vi "2.0.0 Mutation.vi"(8 "error in":errorcluster, 11 "Device Ref in":T1 format="%.0x") -> (0 "error out":errorcluster, 3 "Device Ref out":T1 format="%.0x")   [LabVIEW 2016, in "Ballard Arinc-429 System Explorer.lvlib"]
uses:
  Ballard Arinc-429 System Explorer.lvlib
  <vilib>/NI Veristand/Custom Device API/Custom Device Item Ref.ctl
  NationalInstruments.VeriStand.SystemDefinitionAPI
  Shared/Controls and Global/Global.vi
  <vilib>/NI Veristand/Custom Device Tools/Custom Device Utility Library/NI VeriStand - Search for All Items by GUID.vi
  <vilib>/NI VeriStand/Custom Device Tools/Custom Device Utility Library/Custom Device Utility Library.lvlib
  Shared/Ballard Arinc-429 Shared.lvlib
  <vilib>/NI VeriStand/Custom Device API/Custom Device API.lvlib
  <vilib>/NI Veristand/Custom Device Offline API/Custom Device Offline API.lvlib
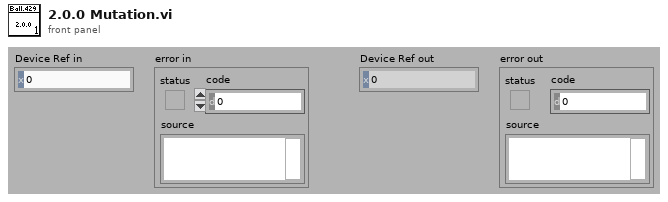
[diagram p1: front panel]
types:
  T1 = typedef "Custom Device API.lvlib/Custom Device Item Ref.ctl" = u64
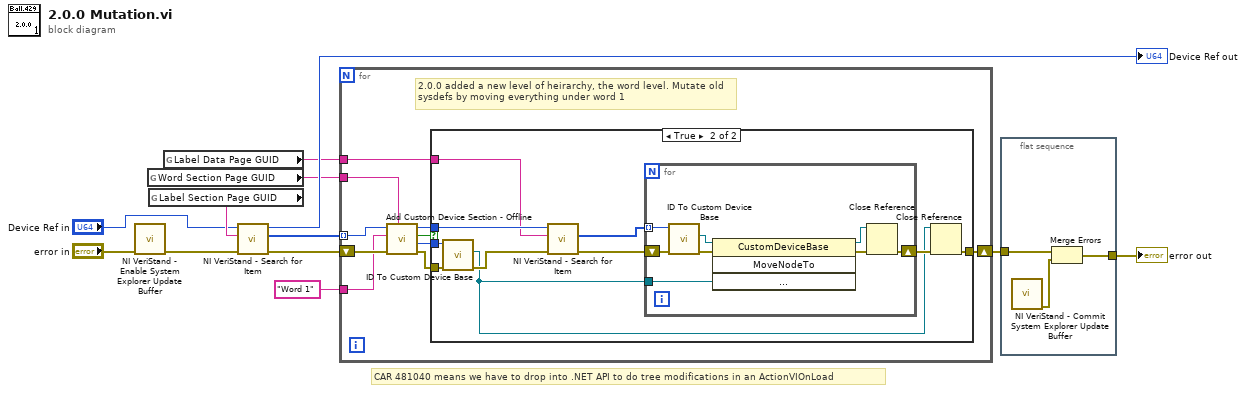
[diagram p0: block diagram]
diagram:
  # "CAR 481040 means we have to drop into .NET API to do tree modifications in an ActionVIOnLoad"
  n1 = call <vilib>:"NI VeriStand - Enable System Explorer Update Buffer.vi"("error in (no error)"="error in") -> ("error out"=w5:errorcluster)  [unwired: 10 in]
  n2 = global read "Global.vi" "Word Section Page GUID"() -> (w7:string)
  n3 = global read "Global.vi" "Label Section Page GUID"() -> (w11:string)
  n4 = global read "Global.vi" "Label Data Page GUID"() -> (w6:string)
  n5 = call-poly <vilib>:"NI VeriStand - Search for Item.vi"("error in"=w5, "Item GUID"=w11, "Section Ref in"="Device Ref in") -> ("error out"=w9:errorcluster, "Item Refs"=w8:T1[], "Section Ref out"=→"Device Ref out":T1)  [unwired: 5 in, 1 out]
  n6 = for {
    shift-right: [w14] -> w3
    shift-left: w9 -> [w22]
    tunnel: w8 -> [w21] mode=indexing
    tunnel: w7 -> [w20]
    tunnel: w6 -> [w18]
    tunnel: "Word 1" ("string") -> [w17]
    # "2.0.0 added a new level of heirarchy, the word level. Mutate old sysdefs by moving everything under word 1"
    n7 = call "Add Custom Device Section - Offline.vi"("GUID (Default Section)"=w20, "error in (no error)"=w22, "Section Name"=w17, "Parent Ref in"=w21) -> ("error out"=w16:errorcluster, "Section Ptr"=w15:T1, "Newly Created?"=w13:bool, "Parent Ref out"=w19:T1)  [unwired: 4 in]
    n8 = case shown="True" w13 {
      tunnel: w19 -> [_ w33]
      tunnel: w18 -> [_ w32]
      tunnel: w16 -> [w23 w29]
      tunnel: w15 -> [_ w27]
      tunnel: [w23 w26] -> w14
      frame False {
        # "There was a beta customer who already has these features so if word 1 exists, ignore it"
      }
      frame True {
        n9 = call <vilib>:"ID To Custom Device Base.vi"("error in (no error)"=w29, "ID in"=w27) -> ("error out"=w28:errorcluster, "BaseNode"=w24:refnum<k24>)  [unwired: 7 in, 1 out]
        n10 = call-poly <vilib>:"NI VeriStand - Search for Item.vi"("error in"=w28, "Item GUID"=w32, "Section Ref in"=w33) -> ("error out"=w31:errorcluster, "Item Refs"=w30:T1[])  [unwired: 5 in, 2 out]
        n11 = for {
          shift-right: [w35] -> w25
          shift-left: w31 -> [w41]
          tunnel: w30 -> [w40] mode=indexing
          tunnel: w24 -> [w36]
          n12 = call <vilib>:"ID To Custom Device Base.vi"("error in (no error)"=w41, "ID in"=w40) -> ("error out"=w39:errorcluster, "BaseNode"=w37:refnum<k24>)  [unwired: 7 in, 1 out]
          n13 = invoke class="CustomDeviceBase" method="MoveNodeTo"(reference=w37, error in=w39, "ParentType"=w36) -> (reference out=w34:refnum<k24>, error out=w38:errorcluster)  [unwired: 1 in, 2 out]
          n14 = Close Reference(reference=w34, error in (no error)=w38) -> (error out=w35:errorcluster)
        }
        n15 = Close Reference(reference=w24, error in (no error)=w25) -> (error out=w26:errorcluster)
      }
    }
  }
  n16 = flat-sequence {
    tunnel: w3 -> [w44]
    tunnel: [w43] -> w2
    frame #0 {
      n17 = call <vilib>:"NI VeriStand - Commit System Explorer Update Buffer.vi"() -> ("error out"=w42:errorcluster)  [unwired: 11 in]
      n18 = Merge Errors(w44, w42) -> (w43:errorcluster)
    }
  }
  "error out" <- w2
